vi "GetChainState.vi"(8 "error in (no error)":errorcluster, 10 "ChainNumber":u8, 11 "ControlState in":T2 {"ChainMask" format="0x%02x"}) -> (0 "error out":errorcluster, 1 "ChainIndex":i32, 2 "ChainState":T1, 3 "ControlState out":T2 {"ChainMask" format="0x%02x"})   [LabVIEW 2023, in "ArduinoSerialBling.lvlib"]
uses:
  ArduinoSerialBling.lvlib
  ControlState.ctl
  ChainState.ctl
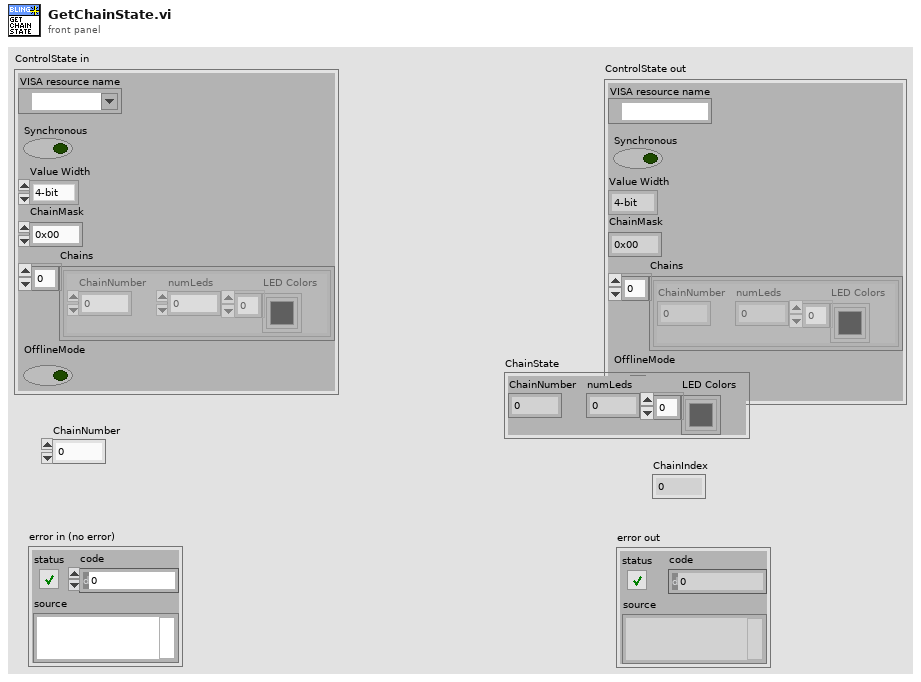
[diagram p1: front panel]
types:
  T1 = typedef "ArduinoSerialBling.lvlib/ChainState.ctl" = cluster{"ChainNumber":u8, "numLeds":u8, "LED Colors":u32[]}
  T2 = typedef "ArduinoSerialBling.lvlib/ControlState.ctl" = cluster{"VISA resource name":refnum<visa-resource-name>, "Synchronous":bool, "Value Width":enum16{"4-bit", "8-bit"}, "ChainMask":u8, "Chains":T1[], "OfflineMode":bool}
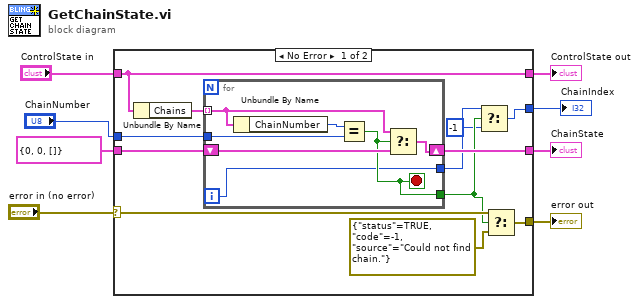
[diagram p0: block diagram]
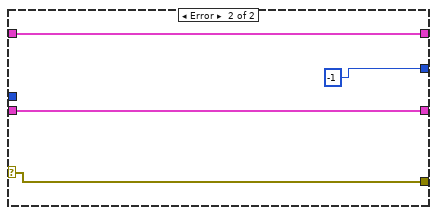
[diagram p2: hidden frame]
diagram:
  n1 = case shown="No Error" "error in (no error)" {
    selector: "error in (no error)" -> [w15 w30]
    tunnel: "ControlState in" -> [w20 w31]
    tunnel: "ChainNumber" -> [w18 _]
    tunnel: [w20 w31] -> w5
    tunnel: [w14 w30] -> w4
    tunnel: [w17 w29] -> w3
    tunnel: T1 {"ChainNumber"=0, "numLeds"=0, "LED Colors"=[]} ("Chain") -> [w16 w29]
    tunnel: [w12 -1 ("f")] -> w1
    frame No Error {
      n2 = Unbundle By Name(w20) -> ("Chains"=w19:T1[])
      n3 = for {
        tunnel: w19 -> [w24] mode=indexing
        tunnel: w18 -> [w26]
        shift-right: [w23] -> w17
        shift-left: w16 -> [w25]
        tunnel: [w22] -> w11
        tunnel: [w21] -> w10
        i -> [w21]
        stop <- w22 stop-if-true
        n4 = Unbundle By Name(w24) -> ("ChainNumber"=w27:u8)
        n5 = Equal?(x=w27, y=w26) -> (x = y?=w22:bool)
        n6 = Select(t=w24, s=w22, f=w25) -> (s? t:f=w23:T1)
      }
      n7 = Select(t=w10, s=w11, f=-1) -> (s? t:f=w12:i32)
      n8 = Select(t=w15, s=w11, f=errorcluster {"status"=TRUE, "code"=-1, "source"="Could not find chain."}) -> (s? t:f=w14:errorcluster)
    }
    frame Error {
    }
  }
  "ControlState out" <- w5
  "error out" <- w4
  "ChainState" <- w3
  "ChainIndex" <- w1
